vi "CommandInOutTest.vi"() -> ()   [LabVIEW 2014, in "examples.lvlib"]
uses:
  examples.lvlib
  vis/tango_vi.llb/fromDevString.vi
  vis/tango_vi.llb/fromDevVarStringArray.vi
  vis/tango_vi.llb/toDevString.vi
  vis/tango_vi.llb/toDevVarStringArray.vi
  vis/tango_vi.llb/fromDevEnum.vi
  vis/tango_vi.llb/toDevShort.vi
  vis/tango_vi.llb/fromDevUShort.vi
  vis/tango_vi.llb/toDevUShort.vi
  vis/tango_vi.llb/fromDevLong.vi
  vis/tango_vi.llb/toDevLong.vi
  vis/tango_vi.llb/fromDevULong.vi
  vis/tango_vi.llb/toDevULong.vi
  vis/tango_vi.llb/fromDevFloat.vi
  vis/tango_vi.llb/toDevFloat.vi
  vis/tango_vi.llb/fromDevDouble.vi
  vis/tango_vi.llb/toDevDouble.vi
  vis/tango_vi.llb/fromDevVarUShortArray.vi
  vis/tango_vi.llb/toDevVarUShortArray.vi
  vis/tango_vi.llb/fromDevVarULongArray.vi
  vis/tango_vi.llb/toDevVarULongArray.vi
  vis/tango_vi.llb/fromDevVarLongArray.vi
  vis/tango_vi.llb/toDevVarLongArray.vi
  vis/tango_vi.llb/fromDevVarShortArray.vi
  vis/tango_vi.llb/toDevVarShortArray.vi
  vis/tango_vi.llb/fromDevVarFloatArray.vi
  vis/tango_vi.llb/toDevVarFloatArray.vi
  vis/tango_vi.llb/fromDevVarDoubleArray.vi
  vis/tango_vi.llb/toDevVarDoubleArray.vi
  vis/tango_vi.llb/fromDevVarCharArray.vi
  vis/tango_vi.llb/toDevVarCharArray.vi
  vis/tango_vi.llb/fromDevVarDoubleStringArray.vi
  vis/tango_vi.llb/toDevVarDoubleStringArray.vi
  vis/tango_vi.llb/fromDevVarLongStringArray.vi
  vis/tango_vi.llb/toDevVarLongStringArray.vi
  vis/tango_vi.llb/fromDevBoolean.vi
  vis/tango_vi.llb/toDevBoolean.vi
  vis/tango_vi.llb/tango.lvlib
panel:
  out "cmd":bool
  out "Void Example":string="DevBoolean"
  out "Graphe déroulant":i32(graph)
  out "TF example":string="DevBoolean"
  out "cmd":bool
  out "data":bool
  out "Argin":bool
  out "Argout":bool
  out "Argin (svalue)":string[](array[string])
  out "Argin (dvalue)":dbl[](array[numeric])=[0.0, 0.0, 0.0, 0.0, 22.0, 144.0, 108.0, 42.0, 254.0, 232.0, 134.0, 30.0, 230.0, 216.0, 161.0, 246.0, 224.0, 86.0, 234.0, 166.0, 49.0, 58.0, 32.0, 211.0, 173.0, 95.0, 77.0, 181.0, 63.0, 73.0, 167.0, 139.0, 214.0, 190.0, 103.0, 103.0, 169.0, 96.0, 65.0, 97.0, 207.0, 72.0, 125.0, 181.0, 232.0, 13.0, 83.0, 114.0, 134.0, 104.0, 222.0, 186.0, 151.0, 6.0, 244.0, 71.0, 19.0, 16.0, 56.0, 155.0, 85.0, 251.0, 65.0, 85.0, 106.0, 68.0, 170.0, 26.0, 143.0, 0.0, 158.0, 43.0, 118.0, 202.0, 61.0, 68.0, 240.0, 57.0, 209.0, 5.0, 98.0, 217.0, 111.0, 7.0, 202.0, 252.0, 200.0, 153.0, 204.0, 237.0, 228.0, 39.0, 81.0, 253.0, 177.0, 126.0, 199.0, 44.0, 36.0, 175.0, 75.0, 209.0, 178.0, 167.0, 71.0, 225.0, 184.0, 2.0, 157.0, 48.0, 226.0, 233.0, 100.0, 110.0, 187.0, 178.0, 2.0, 135.0, 104.0, 251.0, 131.0, 241.0, 155.0, 13.0, 32.0, 205.0, 77.0, 234.0, 75.0, 144.0, 76.0, 162.0, 196.0, 51.0, 92.0, 150.0, 117.0, 79.0, 178.0, 55.0, 131.0, 128.0, 34.0, 21.0, 93.0, 207.0, 230.0, 166.0, 66.0, 107.0, 39.0, 27.0, 201.0, 85.0, 46.0, 15.0, 57.0, 119.0, 112.0, 178.0, 203.0, 181.0, 186.0, 84.0, 144.0, 207.0, 27.0, 215.0, 81.0, 26.0, 153.0, 210.0, 222.0, 175.0, 212.0, 63.0, 227.0, 175.0, 79.0, 219.0, 119.0, 174.0, 36.0, 214.0, 204.0, 213.0, 83.0, 159.0, 255.0, 63.0, 42.0, 236.0, 74.0, 140.0, 119.0, 3.0, 168.0, 232.0, 161.0, 103.0, 146.0, 193.0, 113.0, 1.0, 139.0, 101.0, 51.0, 131.0, 224.0, 211.0, 244.0, 75.0, 119.0, 231.0, 104.0, 41.0, 169.0, 99.0, 112.0, 204.0, 67.0, 210.0, 99.0, 251.0, 141.0, 239.0, 97.0, 144.0, 211.0, 170.0, 68.0, 6.0, 132.0, 235.0, 191.0, 120.0, 102.0, 48.0, 127.0, 1.0, 97.0, 206.0, 9.0, 103.0, 206.0, 167.0, 249.0, 98.0, 74.0, 193.0, 187.0, 30.0, 113.0, 96.0, 73.0, 61.0]
  out "Argout (svalue)":string[](array[string])
  out "Argout (dvalue)":dbl[](array[numeric])=[0.0, 0.0, 0.0, 0.0, 22.0, 144.0, 108.0, 42.0, 254.0, 232.0, 134.0, 30.0, 230.0, 216.0, 161.0, 246.0, 224.0, 86.0, 234.0, 166.0, 49.0, 58.0, 32.0, 211.0, 173.0, 95.0, 77.0, 181.0, 63.0, 73.0, 167.0, 139.0, 214.0, 190.0, 103.0, 103.0, 169.0, 96.0, 65.0, 97.0, 207.0, 72.0, 125.0, 181.0, 232.0, 13.0, 83.0, 114.0, 134.0, 104.0, 222.0, 186.0, 151.0, 6.0, 244.0, 71.0, 19.0, 16.0, 56.0, 155.0, 85.0, 251.0, 65.0, 85.0, 106.0, 68.0, 170.0, 26.0, 143.0, 0.0, 158.0, 43.0, 118.0, 202.0, 61.0, 68.0, 240.0, 57.0, 209.0, 5.0, 98.0, 217.0, 111.0, 7.0, 202.0, 252.0, 200.0, 153.0, 204.0, 237.0, 228.0, 39.0, 81.0, 253.0, 177.0, 126.0, 199.0, 44.0, 36.0, 175.0, 75.0, 209.0, 178.0, 167.0, 71.0, 225.0, 184.0, 2.0, 157.0, 48.0, 226.0, 233.0, 100.0, 110.0, 187.0, 178.0, 2.0, 135.0, 104.0, 251.0, 131.0, 241.0, 155.0, 13.0, 32.0, 205.0, 77.0, 234.0, 75.0, 144.0, 76.0, 162.0, 196.0, 51.0, 92.0, 150.0, 117.0, 79.0, 178.0, 55.0, 131.0, 128.0, 34.0, 21.0, 93.0, 207.0, 230.0, 166.0, 66.0, 107.0, 39.0, 27.0, 201.0, 85.0, 46.0, 15.0, 57.0, 119.0, 112.0, 178.0, 203.0, 181.0, 186.0, 84.0, 144.0, 207.0, 27.0, 215.0, 81.0, 26.0, 153.0, 210.0, 222.0, 175.0, 212.0, 63.0, 227.0, 175.0, 79.0, 219.0, 119.0, 174.0, 36.0, 214.0, 204.0, 213.0, 83.0, 159.0, 255.0, 63.0, 42.0, 236.0, 74.0, 140.0, 119.0, 3.0, 168.0, 232.0, 161.0, 103.0, 146.0, 193.0, 113.0, 1.0, 139.0, 101.0, 51.0, 131.0, 224.0, 211.0, 244.0, 75.0, 119.0, 231.0, 104.0, 41.0, 169.0, 99.0, 112.0, 204.0, 67.0, 210.0, 99.0, 251.0, 141.0, 239.0, 97.0, 144.0, 211.0, 170.0, 68.0, 6.0, 132.0, 235.0, 191.0, 120.0, 102.0, 48.0, 127.0, 1.0, 97.0, 206.0, 9.0, 103.0, 206.0, 167.0, 249.0, 98.0, 74.0, 193.0, 187.0, 30.0, 113.0, 96.0, 73.0, 61.0]
  out "data":bool
  out "cmd":bool
  out "[DBL][String] example":string="DevVarLongStringArray"
  out "[i32][String] example":string="DevVarLongStringArray"
  out "cmd":bool
  out "data":bool
  out "Argout (lvalue)":i32[](array[numeric])=[0, 0, 0, 0, 22, 144, 108, 42, 254, 232, 134, 30, 230, 216, 161, 246, 224, 86, 234, 166, 49, 58, 32, 211, 173, 95, 77, 181, 63, 73, 167, 139, 214, 190, 103, 103, 169, 96, 65, 97, 207, 72, 125, 181, 232, 13, 83, 114, 134, 104, 222, 186, 151, 6, 244, 71, 19, 16, 56, 155, 85, 251, 65, 85, 106, 68, 170, 26, 143, 0, 158, 43, 118, 202, 61, 68, 240, 57, 209, 5, 98, 217, 111, 7, 202, 252, 200, 153, 204, 237, 228, 39, 81, 253, 177, 126, 199, 44, 36, 175, 75, 209, 178, 167, 71, 225, 184, 2, 157, 48, 226, 233, 100, 110, 187, 178, 2, 135, 104, 251, 131, 241, 155, 13, 32, 205, 77, 234, 75, 144, 76, 162, 196, 51, 92, 150, 117, 79, 178, 55, 131, 128, 34, 21, 93, 207, 230, 166, 66, 107, 39, 27, 201, 85, 46, 15, 57, 119, 112, 178, 203, 181, 186, 84, 144, 207, 27, 215, 81, 26, 153, 210, 222, 175, 212, 63, 227, 175, 79, 219, 119, 174, 36, 214, 204, 213, 83, 159, 255, 63, 42, 236, 74, 140, 119, 3, 168, 232, 161, 103, 146, 193, 113, 1, 139, 101, 51, 131, 224, 211, 244, 75, 119, 231, 104, 41, 169, 99, 112, 204, 67, 210, 99, 251, 141, 239, 97, 144, 211, 170, 68, 6, 132, 235, 191, 120, 102, 48, 127, 1, 97, 206, 9, 103, 206, 167, 249, 98, 74, 193, 187, 30, 113, 96, 73, 61]
  out "Argout (svalue)":string[](array[string])
  out "Argin (lvalue)":i32[](array[numeric])=[0, 0, 0, 0, 22, 144, 108, 42, 254, 232, 134, 30, 230, 216, 161, 246, 224, 86, 234, 166, 49, 58, 32, 211, 173, 95, 77, 181, 63, 73, 167, 139, 214, 190, 103, 103, 169, 96, 65, 97, 207, 72, 125, 181, 232, 13, 83, 114, 134, 104, 222, 186, 151, 6, 244, 71, 19, 16, 56, 155, 85, 251, 65, 85, 106, 68, 170, 26, 143, 0, 158, 43, 118, 202, 61, 68, 240, 57, 209, 5, 98, 217, 111, 7, 202, 252, 200, 153, 204, 237, 228, 39, 81, 253, 177, 126, 199, 44, 36, 175, 75, 209, 178, 167, 71, 225, 184, 2, 157, 48, 226, 233, 100, 110, 187, 178, 2, 135, 104, 251, 131, 241, 155, 13, 32, 205, 77, 234, 75, 144, 76, 162, 196, 51, 92, 150, 117, 79, 178, 55, 131, 128, 34, 21, 93, 207, 230, 166, 66, 107, 39, 27, 201, 85, 46, 15, 57, 119, 112, 178, 203, 181, 186, 84, 144, 207, 27, 215, 81, 26, 153, 210, 222, 175, 212, 63, 227, 175, 79, 219, 119, 174, 36, 214, 204, 213, 83, 159, 255, 63, 42, 236, 74, 140, 119, 3, 168, 232, 161, 103, 146, 193, 113, 1, 139, 101, 51, 131, 224, 211, 244, 75, 119, 231, 104, 41, 169, 99, 112, 204, 67, 210, 99, 251, 141, 239, 97, 144, 211, 170, 68, 6, 132, 235, 191, 120, 102, 48, 127, 1, 97, 206, 9, 103, 206, 167, 249, 98, 74, 193, 187, 30, 113, 96, 73, 61]
  out "Argin (svalue)":string[](array[string])
  out "Argout":string[](array[string])
  out "Argin":string[](array[string])
  out "[String] example":string="DevVarStringArray"
  out "cmd":bool
  out "data":bool
  out "Argout":string
  out "Argin":string
  out "data":bool
  out "cmd":bool
  out "String example":string="DevString"
  out "[u8] example":string="DevVarLongArray"
  out "cmd":bool
  out "Argin":u8[](array[numeric])=[0, 0, 89, 52, 22, 144, 108, 42, 254, 232, 134, 30, 230, 216, 161, 246, 224, 86, 234, 166, 49, 58, 32, 211, 173, 95, 77, 181, 63, 73, 167, 139, 214, 190, 103, 103, 169, 96, 65, 97, 207, 72, 125, 181, 232, 13, 83, 114, 134, 104, 222, 186, 151, 6, 244, 71, 19, 16, 56, 155, 85, 251, 65, 85, 106, 68, 170, 26, 143, 0, 158, 43, 118, 202, 61, 68, 240, 57, 209, 5, 98, 217, 111, 7, 202, 252, 200, 153, 204, 237, 228, 39, 81, 253, 177, 126, 199, 44, 36, 175, 75, 209, 178, 167, 71, 225, 184, 2, 157, 48, 226, 233, 100, 110, 187, 178, 2, 135, 104, 251, 131, 241, 155, 13, 32, 205, 77, 234, 75, 144, 76, 162, 196, 51, 92, 150, 117, 79, 178, 55, 131, 128, 34, 21, 93, 207, 230, 166, 66, 107, 39, 27, 201, 85, 46, 15, 57, 119, 112, 178, 203, 181, 186, 84, 144, 207, 27, 215, 81, 26, 153, 210, 222, 175, 212, 63, 227, 175, 79, 219, 119, 174, 36, 214, 204, 213, 83, 159, 255, 63, 42, 236, 74, 140, 119, 3, 168, 232, 161, 103, 146, 193, 113, 1, 139, 101, 51, 131, 224, 211, 244, 75, 119, 231, 104, 41, 169, 99, 112, 204, 67, 210, 99, 251, 141, 239, 97, 144, 211, 170, 68, 6, 132, 235, 191, 120, 102, 48, 127, 1, 97, 206, 9, 103, 206, 167, 249, 98, 74, 193, 187, 30, 113, 96, 73, 61]
  out "Argout":u8[](array[numeric])=[0, 0, 89, 52, 22, 144, 108, 42, 254, 232, 134, 30, 230, 216, 161, 246, 224, 86, 234, 166, 49, 58, 32, 211, 173, 95, 77, 181, 63, 73, 167, 139, 214, 190, 103, 103, 169, 96, 65, 97, 207, 72, 125, 181, 232, 13, 83, 114, 134, 104, 222, 186, 151, 6, 244, 71, 19, 16, 56, 155, 85, 251, 65, 85, 106, 68, 170, 26, 143, 0, 158, 43, 118, 202, 61, 68, 240, 57, 209, 5, 98, 217, 111, 7, 202, 252, 200, 153, 204, 237, 228, 39, 81, 253, 177, 126, 199, 44, 36, 175, 75, 209, 178, 167, 71, 225, 184, 2, 157, 48, 226, 233, 100, 110, 187, 178, 2, 135, 104, 251, 131, 241, 155, 13, 32, 205, 77, 234, 75, 144, 76, 162, 196, 51, 92, 150, 117, 79, 178, 55, 131, 128, 34, 21, 93, 207, 230, 166, 66, 107, 39, 27, 201, 85, 46, 15, 57, 119, 112, 178, 203, 181, 186, 84, 144, 207, 27, 215, 81, 26, 153, 210, 222, 175, 212, 63, 227, 175, 79, 219, 119, 174, 36, 214, 204, 213, 83, 159, 255, 63, 42, 236, 74, 140, 119, 3, 168, 232, 161, 103, 146, 193, 113, 1, 139, 101, 51, 131, 224, 211, 244, 75, 119, 231, 104, 41, 169, 99, 112, 204, 67, 210, 99, 251, 141, 239, 97, 144, 211, 170, 68, 6, 132, 235, 191, 120, 102, 48, 127, 1, 97, 206, 9, 103, 206, 167, 249, 98, 74, 193, 187, 30, 113, 96, 73, 61]
  out "data":bool
  out "[DBL] example":string="DevVarLongArray"
  out "cmd":bool
  out "Argin":dbl[](array[numeric])=[0.0, 0.0, 89.0, 52.0, 22.0, 144.0, 108.0, 42.0, 254.0, 232.0, 134.0, 30.0, 230.0, 216.0, 161.0, 246.0, 224.0, 86.0, 234.0, 166.0, 49.0, 58.0, 32.0, 211.0, 173.0, 95.0, 77.0, 181.0, 63.0, 73.0, 167.0, 139.0, 214.0, 190.0, 103.0, 103.0, 169.0, 96.0, 65.0, 97.0, 207.0, 72.0, 125.0, 181.0, 232.0, 13.0, 83.0, 114.0, 134.0, 104.0, 222.0, 186.0, 151.0, 6.0, 244.0, 71.0, 19.0, 16.0, 56.0, 155.0, 85.0, 251.0, 65.0, 85.0, 106.0, 68.0, 170.0, 26.0, 143.0, 0.0, 158.0, 43.0, 118.0, 202.0, 61.0, 68.0, 240.0, 57.0, 209.0, 5.0, 98.0, 217.0, 111.0, 7.0, 202.0, 252.0, 200.0, 153.0, 204.0, 237.0, 228.0, 39.0, 81.0, 253.0, 177.0, 126.0, 199.0, 44.0, 36.0, 175.0, 75.0, 209.0, 178.0, 167.0, 71.0, 225.0, 184.0, 2.0, 157.0, 48.0, 226.0, 233.0, 100.0, 110.0, 187.0, 178.0, 2.0, 135.0, 104.0, 251.0, 131.0, 241.0, 155.0, 13.0, 32.0, 205.0, 77.0, 234.0, 75.0, 144.0, 76.0, 162.0, 196.0, 51.0, 92.0, 150.0, 117.0, 79.0, 178.0, 55.0, 131.0, 128.0, 34.0, 21.0, 93.0, 207.0, 230.0, 166.0, 66.0, 107.0, 39.0, 27.0, 201.0, 85.0, 46.0, 15.0, 57.0, 119.0, 112.0, 178.0, 203.0, 181.0, 186.0, 84.0, 144.0, 207.0, 27.0, 215.0, 81.0, 26.0, 153.0, 210.0, 222.0, 175.0, 212.0, 63.0, 227.0, 175.0, 79.0, 219.0, 119.0, 174.0, 36.0, 214.0, 204.0, 213.0, 83.0, 159.0, 255.0, 63.0, 42.0, 236.0, 74.0, 140.0, 119.0, 3.0, 168.0, 232.0, 161.0, 103.0, 146.0, 193.0, 113.0, 1.0, 139.0, 101.0, 51.0, 131.0, 224.0, 211.0, 244.0, 75.0, 119.0, 231.0, 104.0, 41.0, 169.0, 99.0, 112.0, 204.0, 67.0, 210.0, 99.0, 251.0, 141.0, 239.0, 97.0, 144.0, 211.0, 170.0, 68.0, 6.0, 132.0, 235.0, 191.0, 120.0, 102.0, 48.0, 127.0, 1.0, 97.0, 206.0, 9.0, 103.0, 206.0, 167.0, 249.0, 98.0, 74.0, 193.0, 187.0, 30.0, 113.0, 96.0, 73.0, 61.0] format="%#_12g"
  out "Argout":dbl[](array[numeric])=[0.0, 0.0, 89.0, 52.0, 22.0, 144.0, 108.0, 42.0, 254.0, 232.0, 134.0, 30.0, 230.0, 216.0, 161.0, 246.0, 224.0, 86.0, 234.0, 166.0, 49.0, 58.0, 32.0, 211.0, 173.0, 95.0, 77.0, 181.0, 63.0, 73.0, 167.0, 139.0, 214.0, 190.0, 103.0, 103.0, 169.0, 96.0, 65.0, 97.0, 207.0, 72.0, 125.0, 181.0, 232.0, 13.0, 83.0, 114.0, 134.0, 104.0, 222.0, 186.0, 151.0, 6.0, 244.0, 71.0, 19.0, 16.0, 56.0, 155.0, 85.0, 251.0, 65.0, 85.0, 106.0, 68.0, 170.0, 26.0, 143.0, 0.0, 158.0, 43.0, 118.0, 202.0, 61.0, 68.0, 240.0, 57.0, 209.0, 5.0, 98.0, 217.0, 111.0, 7.0, 202.0, 252.0, 200.0, 153.0, 204.0, 237.0, 228.0, 39.0, 81.0, 253.0, 177.0, 126.0, 199.0, 44.0, 36.0, 175.0, 75.0, 209.0, 178.0, 167.0, 71.0, 225.0, 184.0, 2.0, 157.0, 48.0, 226.0, 233.0, 100.0, 110.0, 187.0, 178.0, 2.0, 135.0, 104.0, 251.0, 131.0, 241.0, 155.0, 13.0, 32.0, 205.0, 77.0, 234.0, 75.0, 144.0, 76.0, 162.0, 196.0, 51.0, 92.0, 150.0, 117.0, 79.0, 178.0, 55.0, 131.0, 128.0, 34.0, 21.0, 93.0, 207.0, 230.0, 166.0, 66.0, 107.0, 39.0, 27.0, 201.0, 85.0, 46.0, 15.0, 57.0, 119.0, 112.0, 178.0, 203.0, 181.0, 186.0, 84.0, 144.0, 207.0, 27.0, 215.0, 81.0, 26.0, 153.0, 210.0, 222.0, 175.0, 212.0, 63.0, 227.0, 175.0, 79.0, 219.0, 119.0, 174.0, 36.0, 214.0, 204.0, 213.0, 83.0, 159.0, 255.0, 63.0, 42.0, 236.0, 74.0, 140.0, 119.0, 3.0, 168.0, 232.0, 161.0, 103.0, 146.0, 193.0, 113.0, 1.0, 139.0, 101.0, 51.0, 131.0, 224.0, 211.0, 244.0, 75.0, 119.0, 231.0, 104.0, 41.0, 169.0, 99.0, 112.0, 204.0, 67.0, 210.0, 99.0, 251.0, 141.0, 239.0, 97.0, 144.0, 211.0, 170.0, 68.0, 6.0, 132.0, 235.0, 191.0, 120.0, 102.0, 48.0, 127.0, 1.0, 97.0, 206.0, 9.0, 103.0, 206.0, 167.0, 249.0, 98.0, 74.0, 193.0, 187.0, 30.0, 113.0, 96.0, 73.0, 61.0] format="%#_12g"
  out "data":bool
  out "[SGL] example":string="DevVarLongArray"
  out "cmd":bool
  out "Argin":sgl[](array[numeric])=[0.0, 0.0, 89.0, 52.0, 22.0, 144.0, 108.0, 42.0, 254.0, 232.0, 134.0, 30.0, 230.0, 216.0, 161.0, 246.0, 224.0, 86.0, 234.0, 166.0, 49.0, 58.0, 32.0, 211.0, 173.0, 95.0, 77.0, 181.0, 63.0, 73.0, 167.0, 139.0, 214.0, 190.0, 103.0, 103.0, 169.0, 96.0, 65.0, 97.0, 207.0, 72.0, 125.0, 181.0, 232.0, 13.0, 83.0, 114.0, 134.0, 104.0, 222.0, 186.0, 151.0, 6.0, 244.0, 71.0, 19.0, 16.0, 56.0, 155.0, 85.0, 251.0, 65.0, 85.0, 106.0, 68.0, 170.0, 26.0, 143.0, 0.0, 158.0, 43.0, 118.0, 202.0, 61.0, 68.0, 240.0, 57.0, 209.0, 5.0, 98.0, 217.0, 111.0, 7.0, 202.0, 252.0, 200.0, 153.0, 204.0, 237.0, 228.0, 39.0, 81.0, 253.0, 177.0, 126.0, 199.0, 44.0, 36.0, 175.0, 75.0, 209.0, 178.0, 167.0, 71.0, 225.0, 184.0, 2.0, 157.0, 48.0, 226.0, 233.0, 100.0, 110.0, 187.0, 178.0, 2.0, 135.0, 104.0, 251.0, 131.0, 241.0, 155.0, 13.0, 32.0, 205.0, 77.0, 234.0, 75.0, 144.0, 76.0, 162.0, 196.0, 51.0, 92.0, 150.0, 117.0, 79.0, 178.0, 55.0, 131.0, 128.0, 34.0, 21.0, 93.0, 207.0, 230.0, 166.0, 66.0, 107.0, 39.0, 27.0, 201.0, 85.0, 46.0, 15.0, 57.0, 119.0, 112.0, 178.0, 203.0, 181.0, 186.0, 84.0, 144.0, 207.0, 27.0, 215.0, 81.0, 26.0, 153.0, 210.0, 222.0, 175.0, 212.0, 63.0, 227.0, 175.0, 79.0, 219.0, 119.0, 174.0, 36.0, 214.0, 204.0, 213.0, 83.0, 159.0, 255.0, 63.0, 42.0, 236.0, 74.0, 140.0, 119.0, 3.0, 168.0, 232.0, 161.0, 103.0, 146.0, 193.0, 113.0, 1.0, 139.0, 101.0, 51.0, 131.0, 224.0, 211.0, 244.0, 75.0, 119.0, 231.0, 104.0, 41.0, 169.0, 99.0, 112.0, 204.0, 67.0, 210.0, 99.0, 251.0, 141.0, 239.0, 97.0, 144.0, 211.0, 170.0, 68.0, 6.0, 132.0, 235.0, 191.0, 120.0, 102.0, 48.0, 127.0, 1.0, 97.0, 206.0, 9.0, 103.0, 206.0, 167.0, 249.0, 98.0, 74.0, 193.0, 187.0, 30.0, 113.0, 96.0, 73.0, 61.0]
  out "Argout":sgl[](array[numeric])=[0.0, 0.0, 89.0, 52.0, 22.0, 144.0, 108.0, 42.0, 254.0, 232.0, 134.0, 30.0, 230.0, 216.0, 161.0, 246.0, 224.0, 86.0, 234.0, 166.0, 49.0, 58.0, 32.0, 211.0, 173.0, 95.0, 77.0, 181.0, 63.0, 73.0, 167.0, 139.0, 214.0, 190.0, 103.0, 103.0, 169.0, 96.0, 65.0, 97.0, 207.0, 72.0, 125.0, 181.0, 232.0, 13.0, 83.0, 114.0, 134.0, 104.0, 222.0, 186.0, 151.0, 6.0, 244.0, 71.0, 19.0, 16.0, 56.0, 155.0, 85.0, 251.0, 65.0, 85.0, 106.0, 68.0, 170.0, 26.0, 143.0, 0.0, 158.0, 43.0, 118.0, 202.0, 61.0, 68.0, 240.0, 57.0, 209.0, 5.0, 98.0, 217.0, 111.0, 7.0, 202.0, 252.0, 200.0, 153.0, 204.0, 237.0, 228.0, 39.0, 81.0, 253.0, 177.0, 126.0, 199.0, 44.0, 36.0, 175.0, 75.0, 209.0, 178.0, 167.0, 71.0, 225.0, 184.0, 2.0, 157.0, 48.0, 226.0, 233.0, 100.0, 110.0, 187.0, 178.0, 2.0, 135.0, 104.0, 251.0, 131.0, 241.0, 155.0, 13.0, 32.0, 205.0, 77.0, 234.0, 75.0, 144.0, 76.0, 162.0, 196.0, 51.0, 92.0, 150.0, 117.0, 79.0, 178.0, 55.0, 131.0, 128.0, 34.0, 21.0, 93.0, 207.0, 230.0, 166.0, 66.0, 107.0, 39.0, 27.0, 201.0, 85.0, 46.0, 15.0, 57.0, 119.0, 112.0, 178.0, 203.0, 181.0, 186.0, 84.0, 144.0, 207.0, 27.0, 215.0, 81.0, 26.0, 153.0, 210.0, 222.0, 175.0, 212.0, 63.0, 227.0, 175.0, 79.0, 219.0, 119.0, 174.0, 36.0, 214.0, 204.0, 213.0, 83.0, 159.0, 255.0, 63.0, 42.0, 236.0, 74.0, 140.0, 119.0, 3.0, 168.0, 232.0, 161.0, 103.0, 146.0, 193.0, 113.0, 1.0, 139.0, 101.0, 51.0, 131.0, 224.0, 211.0, 244.0, 75.0, 119.0, 231.0, 104.0, 41.0, 169.0, 99.0, 112.0, 204.0, 67.0, 210.0, 99.0, 251.0, 141.0, 239.0, 97.0, 144.0, 211.0, 170.0, 68.0, 6.0, 132.0, 235.0, 191.0, 120.0, 102.0, 48.0, 127.0, 1.0, 97.0, 206.0, 9.0, 103.0, 206.0, 167.0, 249.0, 98.0, 74.0, 193.0, 187.0, 30.0, 113.0, 96.0, 73.0, 61.0]
  out "data":bool
  out "DBL example":string="DevDouble"
  out "cmd":bool
  out "data":bool
  out "Argin":dbl format="%#_30g"
  out "Argout":dbl format="%#_30g"
  out "SGL example":string="DevFloat"
  out "cmd":bool
  out "data":bool
  out "Argin":sgl
  out "Argout":sgl
  out "u32 example":string="DevULong"
  out "cmd":bool
  out "data":bool
  out "Argin":u32
  out "Argout":u32
  out "i32 example":string="DevLong"
  out "cmd":bool
  out "data":bool
  out "Argin":i32
  out "Argout":i32
  out "Argout":u16
  out "Argin":u16
  out "data":bool
  out "cmd":bool
  out "u16 example":string="DevUShort"
  out "Argout":i16
  out "Argin":i16
  out "data":bool
  out "cmd":bool
  out "i16 example":string="DevShort"
  out "[u32] example":string="DevVarLongArray"
  out "cmd":bool
  out "Argin":i32[](array[numeric])=[0, 0, 89, 52, 22, 144, 108, 42, 254, 232, 134, 30, 230, 216, 161, 246, 224, 86, 234, 166, 49, 58, 32, 211, 173, 95, 77, 181, 63, 73, 167, 139, 214, 190, 103, 103, 169, 96, 65, 97, 207, 72, 125, 181, 232, 13, 83, 114, 134, 104, 222, 186, 151, 6, 244, 71, 19, 16, 56, 155, 85, 251, 65, 85, 106, 68, 170, 26, 143, 0, 158, 43, 118, 202, 61, 68, 240, 57, 209, 5, 98, 217, 111, 7, 202, 252, 200, 153, 204, 237, 228, 39, 81, 253, 177, 126, 199, 44, 36, 175, 75, 209, 178, 167, 71, 225, 184, 2, 157, 48, 226, 233, 100, 110, 187, 178, 2, 135, 104, 251, 131, 241, 155, 13, 32, 205, 77, 234, 75, 144, 76, 162, 196, 51, 92, 150, 117, 79, 178, 55, 131, 128, 34, 21, 93, 207, 230, 166, 66, 107, 39, 27, 201, 85, 46, 15, 57, 119, 112, 178, 203, 181, 186, 84, 144, 207, 27, 215, 81, 26, 153, 210, 222, 175, 212, 63, 227, 175, 79, 219, 119, 174, 36, 214, 204, 213, 83, 159, 255, 63, 42, 236, 74, 140, 119, 3, 168, 232, 161, 103, 146, 193, 113, 1, 139, 101, 51, 131, 224, 211, 244, 75, 119, 231, 104, 41, 169, 99, 112, 204, 67, 210, 99, 251, 141, 239, 97, 144, 211, 170, 68, 6, 132, 235, 191, 120, 102, 48, 127, 1, 97, 206, 9, 103, 206, 167, 249, 98, 74, 193, 187, 30, 113, 96, 73, 61]
  out "Argout":u32[](array[numeric])=[0, 0, 89, 52, 22, 144, 108, 42, 254, 232, 134, 30, 230, 216, 161, 246, 224, 86, 234, 166, 49, 58, 32, 211, 173, 95, 77, 181, 63, 73, 167, 139, 214, 190, 103, 103, 169, 96, 65, 97, 207, 72, 125, 181, 232, 13, 83, 114, 134, 104, 222, 186, 151, 6, 244, 71, 19, 16, 56, 155, 85, 251, 65, 85, 106, 68, 170, 26, 143, 0, 158, 43, 118, 202, 61, 68, 240, 57, 209, 5, 98, 217, 111, 7, 202, 252, 200, 153, 204, 237, 228, 39, 81, 253, 177, 126, 199, 44, 36, 175, 75, 209, 178, 167, 71, 225, 184, 2, 157, 48, 226, 233, 100, 110, 187, 178, 2, 135, 104, 251, 131, 241, 155, 13, 32, 205, 77, 234, 75, 144, 76, 162, 196, 51, 92, 150, 117, 79, 178, 55, 131, 128, 34, 21, 93, 207, 230, 166, 66, 107, 39, 27, 201, 85, 46, 15, 57, 119, 112, 178, 203, 181, 186, 84, 144, 207, 27, 215, 81, 26, 153, 210, 222, 175, 212, 63, 227, 175, 79, 219, 119, 174, 36, 214, 204, 213, 83, 159, 255, 63, 42, 236, 74, 140, 119, 3, 168, 232, 161, 103, 146, 193, 113, 1, 139, 101, 51, 131, 224, 211, 244, 75, 119, 231, 104, 41, 169, 99, 112, 204, 67, 210, 99, 251, 141, 239, 97, 144, 211, 170, 68, 6, 132, 235, 191, 120, 102, 48, 127, 1, 97, 206, 9, 103, 206, 167, 249, 98, 74, 193, 187, 30, 113, 96, 73, 61]
  out "data":bool
  out "data":bool
  out "Argout":u16[](array[numeric])=[0, 0, 89, 52, 22, 144, 108, 42, 254, 232, 134, 30, 230, 216, 161, 246, 224, 86, 234, 166, 49, 58, 32, 211, 173, 95, 77, 181, 63, 73, 167, 139, 214, 190, 103, 103, 169, 96, 65, 97, 207, 72, 125, 181, 232, 13, 83, 114, 134, 104, 222, 186, 151, 6, 244, 71, 19, 16, 56, 155, 85, 251, 65, 85, 106, 68, 170, 26, 143, 0, 158, 43, 118, 202, 61, 68, 240, 57, 209, 5, 98, 217, 111, 7, 202, 252, 200, 153, 204, 237, 228, 39, 81, 253, 177, 126, 199, 44, 36, 175, 75, 209, 178, 167, 71, 225, 184, 2, 157, 48, 226, 233, 100, 110, 187, 178, 2, 135, 104, 251, 131, 241, 155, 13, 32, 205, 77, 234, 75, 144, 76, 162, 196, 51, 92, 150, 117, 79, 178, 55, 131, 128, 34, 21, 93, 207, 230, 166, 66, 107, 39, 27, 201, 85, 46, 15, 57, 119, 112, 178, 203, 181, 186, 84, 144, 207, 27, 215, 81, 26, 153, 210, 222, 175, 212, 63, 227, 175, 79, 219, 119, 174, 36, 214, 204, 213, 83, 159, 255, 63, 42, 236, 74, 140, 119, 3, 168, 232, 161, 103, 146, 193, 113, 1, 139, 101, 51, 131, 224, 211, 244, 75, 119, 231, 104, 41, 169, 99, 112, 204, 67, 210, 99, 251, 141, 239, 97, 144, 211, 170, 68, 6, 132, 235, 191, 120, 102, 48, 127, 1, 97, 206, 9, 103, 206, 167, 249, 98, 74, 193, 187, 30, 113, 96, 73, 61]
  out "Argin":u16[](array[numeric])=[0, 0, 89, 52, 22, 144, 108, 42, 254, 232, 134, 30, 230, 216, 161, 246, 224, 86, 234, 166, 49, 58, 32, 211, 173, 95, 77, 181, 63, 73, 167, 139, 214, 190, 103, 103, 169, 96, 65, 97, 207, 72, 125, 181, 232, 13, 83, 114, 134, 104, 222, 186, 151, 6, 244, 71, 19, 16, 56, 155, 85, 251, 65, 85, 106, 68, 170, 26, 143, 0, 158, 43, 118, 202, 61, 68, 240, 57, 209, 5, 98, 217, 111, 7, 202, 252, 200, 153, 204, 237, 228, 39, 81, 253, 177, 126, 199, 44, 36, 175, 75, 209, 178, 167, 71, 225, 184, 2, 157, 48, 226, 233, 100, 110, 187, 178, 2, 135, 104, 251, 131, 241, 155, 13, 32, 205, 77, 234, 75, 144, 76, 162, 196, 51, 92, 150, 117, 79, 178, 55, 131, 128, 34, 21, 93, 207, 230, 166, 66, 107, 39, 27, 201, 85, 46, 15, 57, 119, 112, 178, 203, 181, 186, 84, 144, 207, 27, 215, 81, 26, 153, 210, 222, 175, 212, 63, 227, 175, 79, 219, 119, 174, 36, 214, 204, 213, 83, 159, 255, 63, 42, 236, 74, 140, 119, 3, 168, 232, 161, 103, 146, 193, 113, 1, 139, 101, 51, 131, 224, 211, 244, 75, 119, 231, 104, 41, 169, 99, 112, 204, 67, 210, 99, 251, 141, 239, 97, 144, 211, 170, 68, 6, 132, 235, 191, 120, 102, 48, 127, 1, 97, 206, 9, 103, 206, 167, 249, 98, 74, 193, 187, 30, 113, 96, 73, 61]
  out "cmd":bool
  out "[u16] example":string="DevVarLongArray"
  out "data":bool
  out "Argout":i16[](array[numeric])=[0, 0, 89, 52, 22, 144, 108, 42, 254, 232, 134, 30, 230, 216, 161, 246, 224, 86, 234, 166, 49, 58, 32, 211, 173, 95, 77, 181, 63, 73, 167, 139, 214, 190, 103, 103, 169, 96, 65, 97, 207, 72, 125, 181, 232, 13, 83, 114, 134, 104, 222, 186, 151, 6, 244, 71, 19, 16, 56, 155, 85, 251, 65, 85, 106, 68, 170, 26, 143, 0, 158, 43, 118, 202, 61, 68, 240, 57, 209, 5, 98, 217, 111, 7, 202, 252, 200, 153, 204, 237, 228, 39, 81, 253, 177, 126, 199, 44, 36, 175, 75, 209, 178, 167, 71, 225, 184, 2, 157, 48, 226, 233, 100, 110, 187, 178, 2, 135, 104, 251, 131, 241, 155, 13, 32, 205, 77, 234, 75, 144, 76, 162, 196, 51, 92, 150, 117, 79, 178, 55, 131, 128, 34, 21, 93, 207, 230, 166, 66, 107, 39, 27, 201, 85, 46, 15, 57, 119, 112, 178, 203, 181, 186, 84, 144, 207, 27, 215, 81, 26, 153, 210, 222, 175, 212, 63, 227, 175, 79, 219, 119, 174, 36, 214, 204, 213, 83, 159, 255, 63, 42, 236, 74, 140, 119, 3, 168, 232, 161, 103, 146, 193, 113, 1, 139, 101, 51, 131, 224, 211, 244, 75, 119, 231, 104, 41, 169, 99, 112, 204, 67, 210, 99, 251, 141, 239, 97, 144, 211, 170, 68, 6, 132, 235, 191, 120, 102, 48, 127, 1, 97, 206, 9, 103, 206, 167, 249, 98, 74, 193, 187, 30, 113, 96, 73, 61]
  out "Argin":i32[](array[numeric])=[0, 0, 89, 52, 22, 144, 108, 42, 254, 232, 134, 30, 230, 216, 161, 246, 224, 86, 234, 166, 49, 58, 32, 211, 173, 95, 77, 181, 63, 73, 167, 139, 214, 190, 103, 103, 169, 96, 65, 97, 207, 72, 125, 181, 232, 13, 83, 114, 134, 104, 222, 186, 151, 6, 244, 71, 19, 16, 56, 155, 85, 251, 65, 85, 106, 68, 170, 26, 143, 0, 158, 43, 118, 202, 61, 68, 240, 57, 209, 5, 98, 217, 111, 7, 202, 252, 200, 153, 204, 237, 228, 39, 81, 253, 177, 126, 199, 44, 36, 175, 75, 209, 178, 167, 71, 225, 184, 2, 157, 48, 226, 233, 100, 110, 187, 178, 2, 135, 104, 251, 131, 241, 155, 13, 32, 205, 77, 234, 75, 144, 76, 162, 196, 51, 92, 150, 117, 79, 178, 55, 131, 128, 34, 21, 93, 207, 230, 166, 66, 107, 39, 27, 201, 85, 46, 15, 57, 119, 112, 178, 203, 181, 186, 84, 144, 207, 27, 215, 81, 26, 153, 210, 222, 175, 212, 63, 227, 175, 79, 219, 119, 174, 36, 214, 204, 213, 83, 159, 255, 63, 42, 236, 74, 140, 119, 3, 168, 232, 161, 103, 146, 193, 113, 1, 139, 101, 51, 131, 224, 211, 244, 75, 119, 231, 104, 41, 169, 99, 112, 204, 67, 210, 99, 251, 141, 239, 97, 144, 211, 170, 68, 6, 132, 235, 191, 120, 102, 48, 127, 1, 97, 206, 9, 103, 206, 167, 249, 98, 74, 193, 187, 30, 113, 96, 73, 61]
  out "cmd":bool
  out "[i16] example":string="DevVarLongArray"
  out "data":bool
  out "Argout":i32[](array[numeric])=[0, 0, 89, 52, 22, 144, 108, 42, 254, 232, 134, 30, 230, 216, 161, 246, 224, 86, 234, 166, 49, 58, 32, 211, 173, 95, 77, 181, 63, 73, 167, 139, 214, 190, 103, 103, 169, 96, 65, 97, 207, 72, 125, 181, 232, 13, 83, 114, 134, 104, 222, 186, 151, 6, 244, 71, 19, 16, 56, 155, 85, 251, 65, 85, 106, 68, 170, 26, 143, 0, 158, 43, 118, 202, 61, 68, 240, 57, 209, 5, 98, 217, 111, 7, 202, 252, 200, 153, 204, 237, 228, 39, 81, 253, 177, 126, 199, 44, 36, 175, 75, 209, 178, 167, 71, 225, 184, 2, 157, 48, 226, 233, 100, 110, 187, 178, 2, 135, 104, 251, 131, 241, 155, 13, 32, 205, 77, 234, 75, 144, 76, 162, 196, 51, 92, 150, 117, 79, 178, 55, 131, 128, 34, 21, 93, 207, 230, 166, 66, 107, 39, 27, 201, 85, 46, 15, 57, 119, 112, 178, 203, 181, 186, 84, 144, 207, 27, 215, 81, 26, 153, 210, 222, 175, 212, 63, 227, 175, 79, 219, 119, 174, 36, 214, 204, 213, 83, 159, 255, 63, 42, 236, 74, 140, 119, 3, 168, 232, 161, 103, 146, 193, 113, 1, 139, 101, 51, 131, 224, 211, 244, 75, 119, 231, 104, 41, 169, 99, 112, 204, 67, 210, 99, 251, 141, 239, 97, 144, 211, 170, 68, 6, 132, 235, 191, 120, 102, 48, 127, 1, 97, 206, 9, 103, 206, 167, 249, 98, 74, 193, 187, 30, 113, 96, 73, 61]
  out "Argin":i32[](array[numeric])=[0, 0, 89, 52, 22, 144, 108, 42, 254, 232, 134, 30, 230, 216, 161, 246, 224, 86, 234, 166, 49, 58, 32, 211, 173, 95, 77, 181, 63, 73, 167, 139, 214, 190, 103, 103, 169, 96, 65, 97, 207, 72, 125, 181, 232, 13, 83, 114, 134, 104, 222, 186, 151, 6, 244, 71, 19, 16, 56, 155, 85, 251, 65, 85, 106, 68, 170, 26, 143, 0, 158, 43, 118, 202, 61, 68, 240, 57, 209, 5, 98, 217, 111, 7, 202, 252, 200, 153, 204, 237, 228, 39, 81, 253, 177, 126, 199, 44, 36, 175, 75, 209, 178, 167, 71, 225, 184, 2, 157, 48, 226, 233, 100, 110, 187, 178, 2, 135, 104, 251, 131, 241, 155, 13, 32, 205, 77, 234, 75, 144, 76, 162, 196, 51, 92, 150, 117, 79, 178, 55, 131, 128, 34, 21, 93, 207, 230, 166, 66, 107, 39, 27, 201, 85, 46, 15, 57, 119, 112, 178, 203, 181, 186, 84, 144, 207, 27, 215, 81, 26, 153, 210, 222, 175, 212, 63, 227, 175, 79, 219, 119, 174, 36, 214, 204, 213, 83, 159, 255, 63, 42, 236, 74, 140, 119, 3, 168, 232, 161, 103, 146, 193, 113, 1, 139, 101, 51, 131, 224, 211, 244, 75, 119, 231, 104, 41, 169, 99, 112, 204, 67, 210, 99, 251, 141, 239, 97, 144, 211, 170, 68, 6, 132, 235, 191, 120, 102, 48, 127, 1, 97, 206, 9, 103, 206, 167, 249, 98, 74, 193, 187, 30, 113, 96, 73, 61]
  out "cmd":bool
  out "[I32] example":string="DevVarLongArray"
  out "alive":bool
  out "State Color":u32(colorbox)=16448250
  out "Status":string
  out "State String":string
  out "State Code":i16
  in  "TangoTest Device Name":string="sys/tg_test/1"
  # "TANGO  Binding for LabVIEW - Command I/O example"
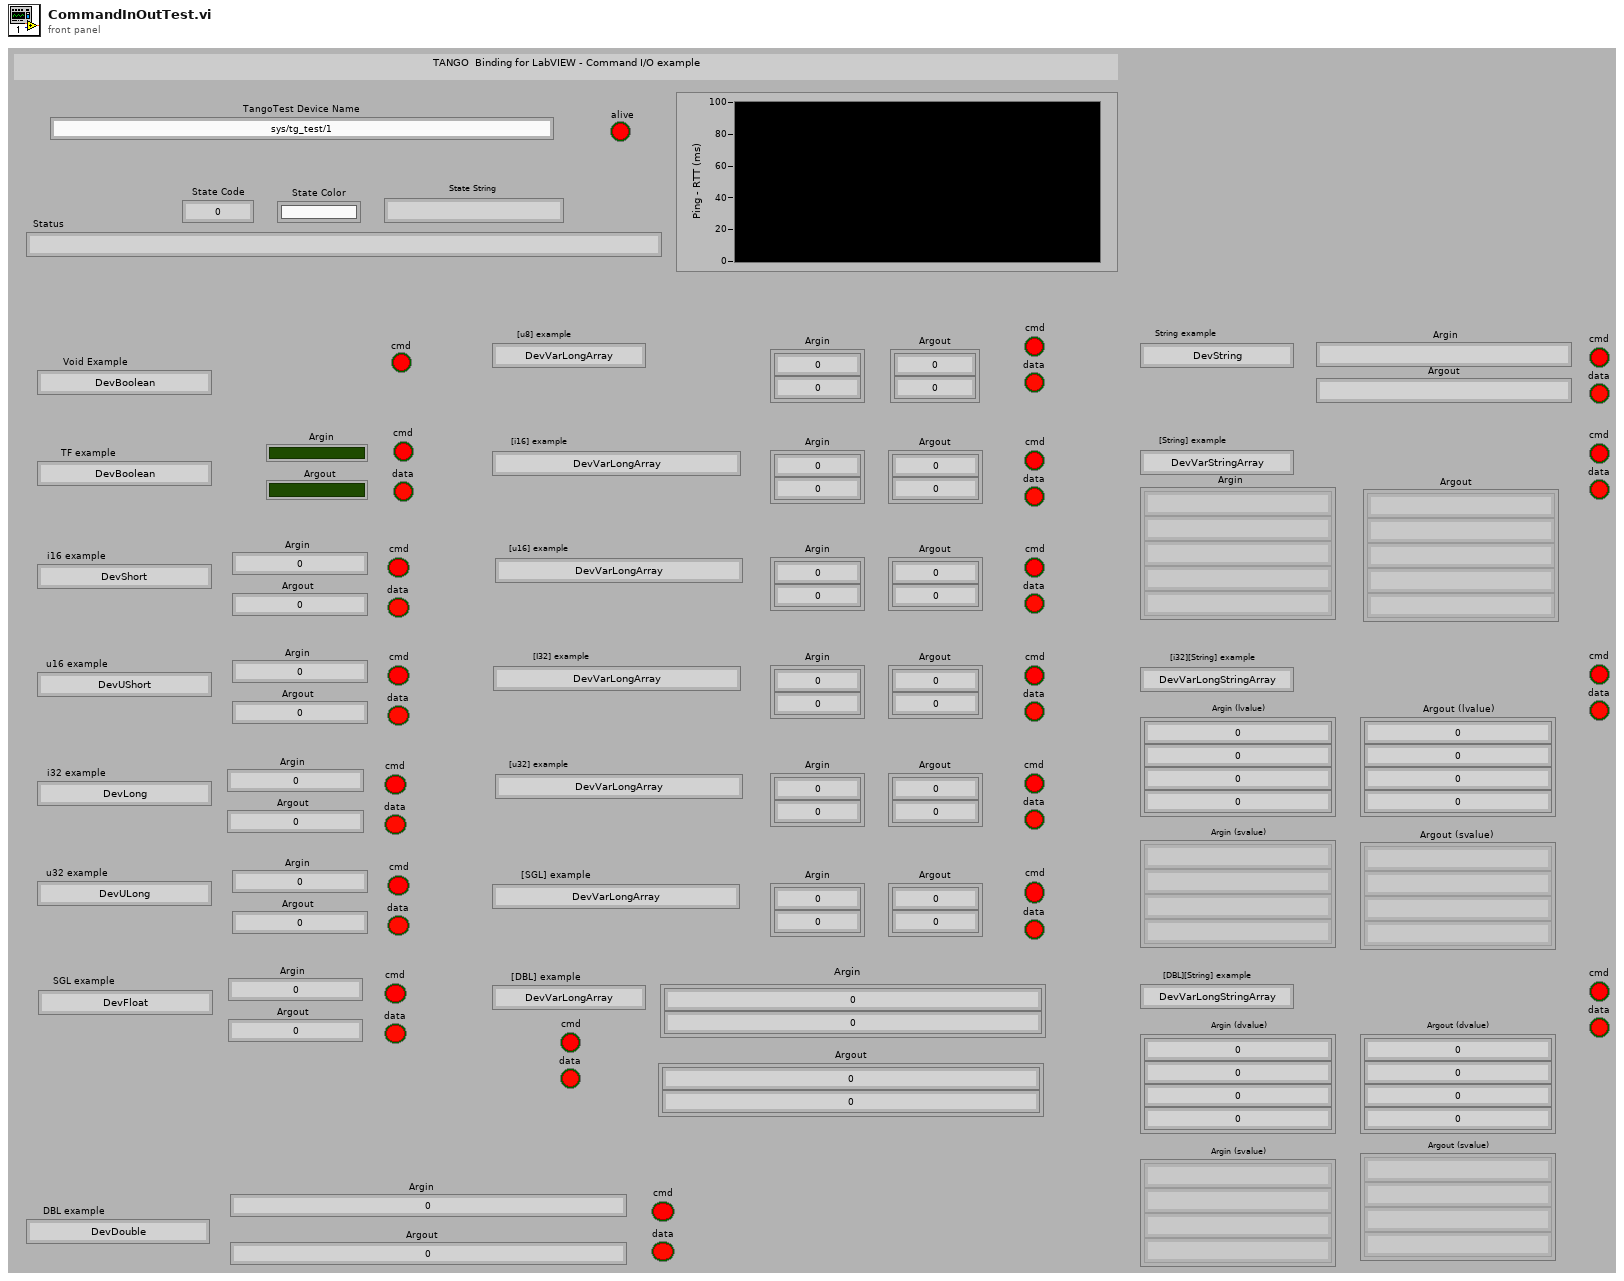
[diagram p1: front panel]
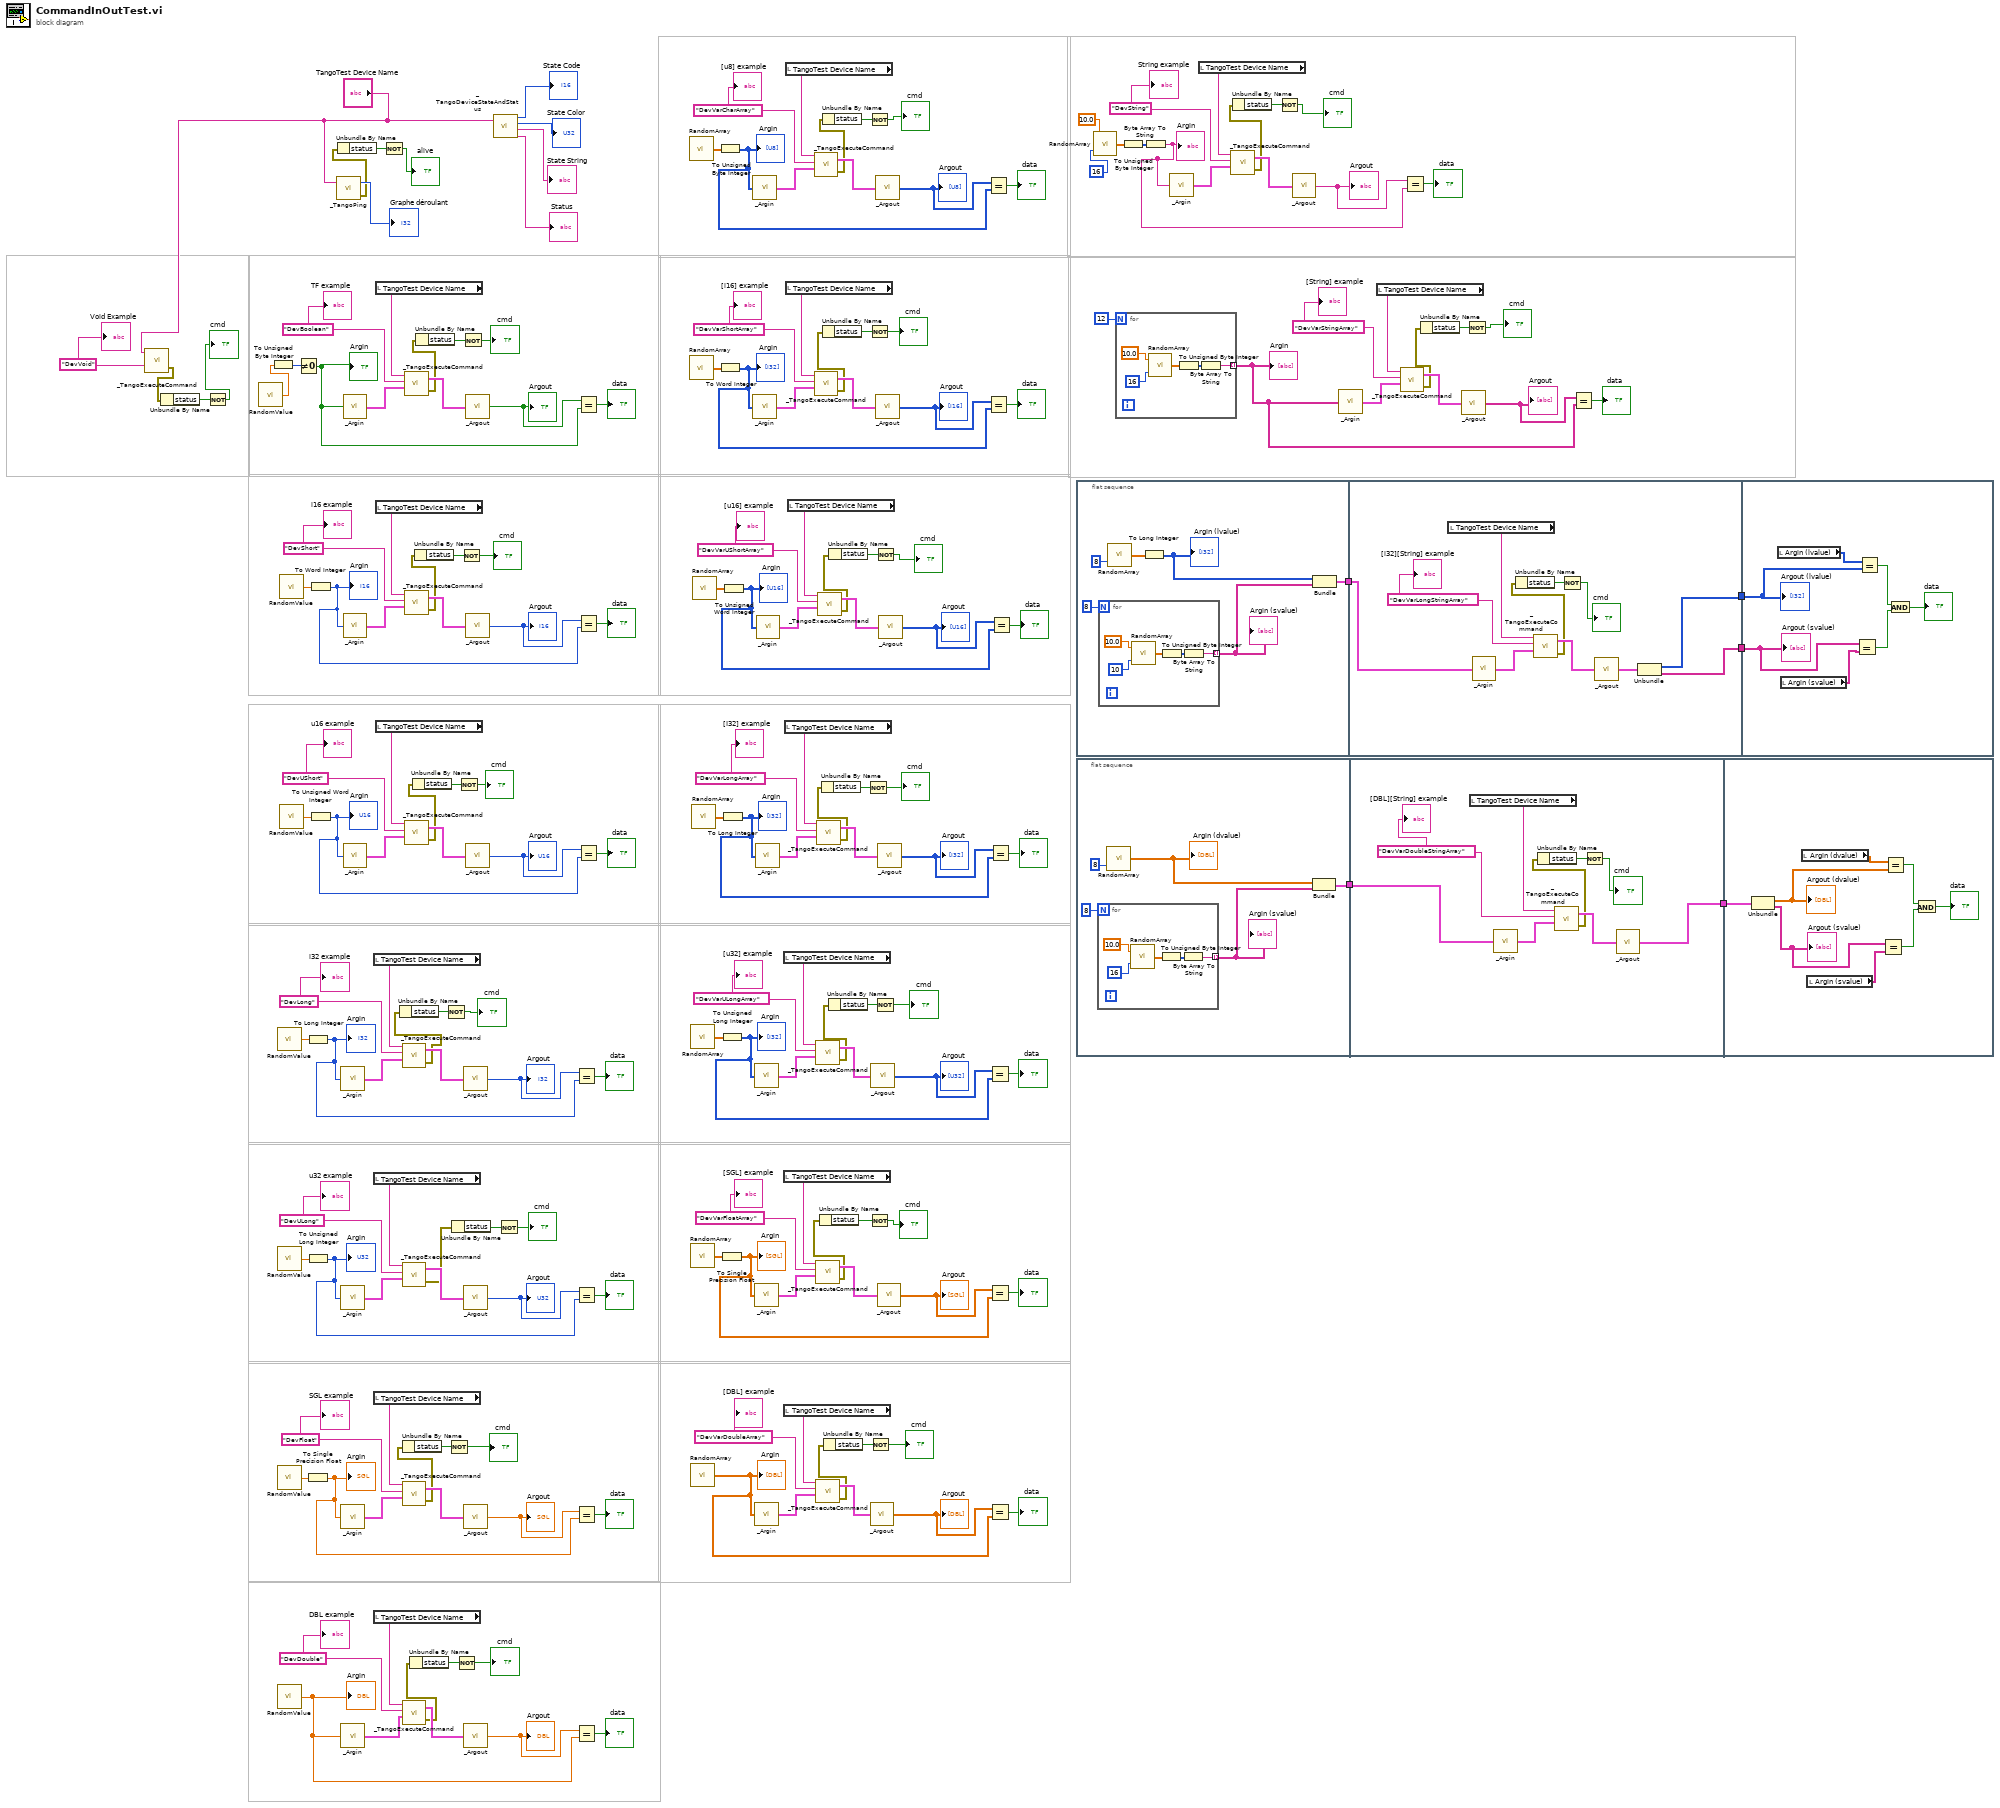
[diagram p0: block diagram]
diagram:
  w59 = "DevVoid"
  w70 = "DevBoolean"
  w80 = "DevVarStringArray"
  w88 = "DevVarCharArray"
  w98 = "DevVarDoubleArray"
  w107 = "DevVarFloatArray"
  w113 = "DevDouble"
  w116 = "DevFloat"
  w127 = "DevULong"
  w133 = "DevLong"
  w144 = "DevUShort"
  w152 = "DevShort"
  w157 = "DevVarULongArray"
  w168 = "DevVarUShortArray"
  w176 = "DevVarShortArray"
  w182 = "DevString"
  w190 = "DevVarLongArray"
  n1 = call "_TangoExecuteCommand.vi"("command name"=w59, "device name"="TangoTest Device Name") -> ("error out"=w52:errorcluster)  [unwired: 2 in, 1 out]
  n2 = Unbundle By Name(w52) -> ("status"=w53:bool)
  n3 = Not(x=w53) -> (.not. x?=→"cmd":bool)
  n4 = call "RandomValue.vi"() -> ("random value"=w1:dbl)  [unwired: 1 in]
  n5 = To Unsigned Byte Integer(number=w1) -> (unsigned 8bit integer=w67:u8)
  n6 = call "RandomValue.vi"() -> ("random value"=w135:dbl)  [unwired: 1 in]
  n7 = call "RandomValue.vi"() -> ("random value"=w125:dbl)  [unwired: 1 in]
  n8 = call "RandomValue.vi"() -> ("random value"=w118:dbl)  [unwired: 1 in]
  n9 = call "RandomValue.vi"() -> ("random value"=w2:dbl)  [unwired: 1 in]
  "Argin" <- w2
  n10 = call "RandomValue.vi"() -> ("random value"=w150:dbl)  [unwired: 1 in]
  n11 = call "RandomValue.vi"() -> ("random value"=w142:dbl)  [unwired: 1 in]
  n12 = Not Equal To 0?(x=w67) -> (x != 0?=w66:bool)
  "Argin" <- w66
  n13 = To Long Integer(number=w135) -> (32bit integer=w138:i32)
  "Argin" <- w138
  n14 = To Unsigned Long Integer(number=w125) -> (unsigned 32bit integer=w122:u32)
  "Argin" <- w122
  n15 = To Single Precision Float(number=w118) -> (single precision float=w121:sgl)
  "Argin" <- w121
  n16 = To Word Integer(number=w150) -> (16bit integer=w148:i16)
  "Argin" <- w148
  n17 = To Unsigned Word Integer(number=w142) -> (unsigned 16bit integer=w139:u16)
  "Argin" <- w139
  n18 = call "_TangoPing.vi"("device name"="TangoTest Device Name") -> ("error out"=w4:errorcluster, "rrt"=→"Graphe déroulant":i32)  [unwired: 1 in]
  n19 = Unbundle By Name(w4) -> ("status"=w5:bool)
  n20 = call-poly "_Argin.vi"("argin"=w138) -> ("ArgIO"=w131:cluster{"num data":u8[], "str data":string[]})
  n21 = call-poly "_Argin.vi"("argin"=w122) -> ("ArgIO"=w130:cluster{"num data":u8[], "str data":string[]})
  n22 = call-poly "_Argin.vi"("argin"=w121) -> ("ArgIO"=w114:cluster{"num data":u8[], "str data":string[]})
  n23 = call-poly "_Argin.vi"("argin"=w2) -> ("ArgIO"=w57:cluster{"num data":u8[], "str data":string[]})
  n24 = call-poly "_Argin.vi"("argin"=w66) -> ("ArgIO"=w68:cluster{"num data":u8[], "str data":string[]})
  n25 = call-poly "_Argin.vi"("argin"=w148) -> ("ArgIO"=w154:cluster{"num data":u8[], "str data":string[]})
  n26 = call-poly "_Argin.vi"("argin"=w139) -> ("ArgIO"=w146:cluster{"num data":u8[], "str data":string[]})
  n27 = local read "TangoTest Device Name"() -> (w134:string)
  n28 = local read "TangoTest Device Name"() -> (w126:string)
  n29 = local read "TangoTest Device Name"() -> (w117:string)
  n30 = local read "TangoTest Device Name"() -> (w112:string)
  n31 = local read "TangoTest Device Name"() -> (w71:string)
  n32 = local read "TangoTest Device Name"() -> (w151:string)
  n33 = local read "TangoTest Device Name"() -> (w143:string)
  n34 = Not(x=w5) -> (.not. x?=→"alive":bool)
  n35 = call "_TangoExecuteCommand.vi"("argin"=w131, "command name"=w133, "device name"=w134) -> ("error out"=w39:errorcluster, "argout"=w132:cluster{"num data":u8[], "str data":string[]})  [unwired: 1 in]
  n36 = Unbundle By Name(w39) -> ("status"=w41:bool)
  n37 = call "_TangoExecuteCommand.vi"("argin"=w130, "command name"=w127, "device name"=w126) -> ("error out"=w128:errorcluster, "argout"=w129:cluster{"num data":u8[], "str data":string[]})  [unwired: 1 in]
  n38 = call "_TangoExecuteCommand.vi"("argin"=w114, "command name"=w116, "device name"=w117) -> ("error out"=w36:errorcluster, "argout"=w115:cluster{"num data":u8[], "str data":string[]})  [unwired: 1 in]
  n39 = Unbundle By Name(w36) -> ("status"=w38:bool)
  n40 = call "_TangoExecuteCommand.vi"("argin"=w57, "command name"=w113, "device name"=w112) -> ("error out"=w33:errorcluster, "argout"=w56:cluster{"num data":u8[], "str data":string[]})  [unwired: 1 in]
  n41 = call "_TangoExecuteCommand.vi"("argin"=w68, "command name"=w70, "device name"=w71) -> ("error out"=w48:errorcluster, "argout"=w69:cluster{"num data":u8[], "str data":string[]})  [unwired: 1 in]
  n42 = call "_TangoExecuteCommand.vi"("argin"=w154, "command name"=w152, "device name"=w151) -> ("error out"=w45:errorcluster, "argout"=w153:cluster{"num data":u8[], "str data":string[]})  [unwired: 1 in]
  n43 = call "_TangoExecuteCommand.vi"("argin"=w146, "command name"=w144, "device name"=w143) -> ("error out"=w42:errorcluster, "argout"=w145:cluster{"num data":u8[], "str data":string[]})  [unwired: 1 in]
  n44 = Unbundle By Name(w33) -> ("status"=w35:bool)
  n45 = Unbundle By Name(w42) -> ("status"=w44:bool)
  n46 = Unbundle By Name(w45) -> ("status"=w47:bool)
  n47 = Unbundle By Name(w48) -> ("status"=w50:bool)
  n48 = Not(x=w41) -> (.not. x?=→"cmd":bool)
  n49 = Not(x=w38) -> (.not. x?=→"cmd":bool)
  n50 = Unbundle By Name(w128) -> ("status"=w55:bool)
  n51 = Not(x=w35) -> (.not. x?=→"cmd":bool)
  n52 = Not(x=w44) -> (.not. x?=→"cmd":bool)
  n53 = Not(x=w47) -> (.not. x?=→"cmd":bool)
  n54 = Not(x=w50) -> (.not. x?=→"cmd":bool)
  n55 = call-poly "_Argout.vi"("ArgIO"=w132) -> ("argout"=w137:i32)
  "Argout" <- w137
  n56 = call-poly "_Argout.vi"("ArgIO"=w129) -> ("argout"=w123:u32)
  "Argout" <- w123
  n57 = call-poly "_Argout.vi"("ArgIO"=w115) -> ("argout"=w120:sgl)
  "Argout" <- w120
  n58 = call-poly "_Argout.vi"("ArgIO"=w56) -> ("argout"=w110:dbl)
  "Argout" <- w110
  n59 = call-poly "_Argout.vi"("ArgIO"=w69) -> ("argout"=w73:bool)
  "Argout" <- w73
  n60 = call-poly "_Argout.vi"("ArgIO"=w153) -> ("argout"=w147:i16)
  "Argout" <- w147
  n61 = call-poly "_Argout.vi"("ArgIO"=w145) -> ("argout"=w140:u16)
  "Argout" <- w140
  n62 = call "_TangoDeviceStateAndStatus.vi"("Device Name"="TangoTest Device Name") -> ("Status"=→"Status":string, "State String"=→"State String":string, "State Color"=→"State Color":u32, "State Code"=→"State Code":i16)  [unwired: 1 in, 1 out]
  n63 = Not(x=w55) -> (.not. x?=→"cmd":bool)
  n64 = Equal?(x=w137, y=w138) -> (x = y?=→"data":bool)
  n65 = Equal?(x=w123, y=w122) -> (x = y?=→"data":bool)
  n66 = Equal?(x=w120, y=w121) -> (x = y?=→"data":bool)
  n67 = Equal?(x=w110, y=w2) -> (x = y?=→"data":bool)
  n68 = Equal?(x=w73, y=w66) -> (x = y?=→"data":bool)
  n69 = Equal?(x=w147, y=w148) -> (x = y?=→"data":bool)
  n70 = Equal?(x=w140, y=w139) -> (x = y?=→"data":bool)
  n71 = call "RandomArray.vi"() -> ("random array"=w90:dbl[])  [unwired: 2 in]
  n72 = call "RandomArray.vi"() -> ("random array"=w174:dbl[])  [unwired: 2 in]
  n73 = call "RandomArray.vi"() -> ("random array"=w159:dbl[])  [unwired: 2 in]
  n74 = call "RandomArray.vi"() -> ("random array"=w105:dbl[])  [unwired: 2 in]
  n75 = call "RandomArray.vi"() -> ("random array"=w95:dbl[])  [unwired: 2 in]
  "Argin" <- w95
  n76 = call "RandomArray.vi"() -> ("random array"=w188:dbl[])  [unwired: 2 in]
  n77 = call "RandomArray.vi"() -> ("random array"=w166:dbl[])  [unwired: 2 in]
  n78 = To Unsigned Byte Integer(number=w90) -> (unsigned 8bit integer=w91:u8[])
  "Argin" <- w91
  n79 = To Word Integer(number=w174) -> (16bit integer=w173:i16[])
  "Argin" <- w173
  n80 = To Unsigned Long Integer(number=w159) -> (unsigned 32bit integer=w160:u32[])
  "Argin" <- w160
  n81 = To Single Precision Float(number=w105) -> (single precision float=w104:sgl[])
  "Argin" <- w104
  n82 = To Long Integer(number=w188) -> (32bit integer=w187:i32[])
  "Argin" <- w187
  n83 = To Unsigned Word Integer(number=w166) -> (unsigned 16bit integer=w165:u16[])
  "Argin" <- w165
  n84 = call-poly "_Argin.vi"("argin"=w91) -> ("ArgIO"=w87:cluster{"num data":u8[], "str data":string[]})
  n85 = call-poly "_Argin.vi"("argin"=w173) -> ("ArgIO"=w178:cluster{"num data":u8[], "str data":string[]})
  n86 = call-poly "_Argin.vi"("argin"=w160) -> ("ArgIO"=w155:cluster{"num data":u8[], "str data":string[]})
  n87 = call-poly "_Argin.vi"("argin"=w104) -> ("ArgIO"=w109:cluster{"num data":u8[], "str data":string[]})
  n88 = call-poly "_Argin.vi"("argin"=w95) -> ("ArgIO"=w96:cluster{"num data":u8[], "str data":string[]})
  n89 = call-poly "_Argin.vi"("argin"=w187) -> ("ArgIO"=w192:cluster{"num data":u8[], "str data":string[]})
  n90 = call-poly "_Argin.vi"("argin"=w165) -> ("ArgIO"=w170:cluster{"num data":u8[], "str data":string[]})
  n91 = local read "TangoTest Device Name"() -> (w158:string)
  n92 = local read "TangoTest Device Name"() -> (w106:string)
  n93 = local read "TangoTest Device Name"() -> (w99:string)
  n94 = local read "TangoTest Device Name"() -> (w189:string)
  n95 = local read "TangoTest Device Name"() -> (w89:string)
  n96 = local read "TangoTest Device Name"() -> (w175:string)
  n97 = local read "TangoTest Device Name"() -> (w167:string)
  n98 = call "_TangoExecuteCommand.vi"("argin"=w87, "command name"=w88, "device name"=w89) -> ("error out"=w12:errorcluster, "argout"=w60:cluster{"num data":u8[], "str data":string[]})  [unwired: 1 in]
  n99 = call "_TangoExecuteCommand.vi"("argin"=w178, "command name"=w176, "device name"=w175) -> ("error out"=w15:errorcluster, "argout"=w177:cluster{"num data":u8[], "str data":string[]})  [unwired: 1 in]
  n100 = call "_TangoExecuteCommand.vi"("argin"=w155, "command name"=w157, "device name"=w158) -> ("error out"=w24:errorcluster, "argout"=w156:cluster{"num data":u8[], "str data":string[]})  [unwired: 1 in]
  n101 = call "_TangoExecuteCommand.vi"("argin"=w109, "command name"=w107, "device name"=w106) -> ("error out"=w27:errorcluster, "argout"=w108:cluster{"num data":u8[], "str data":string[]})  [unwired: 1 in]
  n102 = call "_TangoExecuteCommand.vi"("argin"=w96, "command name"=w98, "device name"=w99) -> ("error out"=w30:errorcluster, "argout"=w97:cluster{"num data":u8[], "str data":string[]})  [unwired: 1 in]
  n103 = call "_TangoExecuteCommand.vi"("argin"=w192, "command name"=w190, "device name"=w189) -> ("error out"=w21:errorcluster, "argout"=w191:cluster{"num data":u8[], "str data":string[]})  [unwired: 1 in]
  n104 = call "_TangoExecuteCommand.vi"("argin"=w170, "command name"=w168, "device name"=w167) -> ("error out"=w19:errorcluster, "argout"=w169:cluster{"num data":u8[], "str data":string[]})  [unwired: 1 in]
  n105 = Unbundle By Name(w27) -> ("status"=w29:bool)
  n106 = Unbundle By Name(w21) -> ("status"=w23:bool)
  n107 = Unbundle By Name(w12) -> ("status"=w14:bool)
  n108 = Unbundle By Name(w15) -> ("status"=w17:bool)
  n109 = Unbundle By Name(w30) -> ("status"=w32:bool)
  n110 = Unbundle By Name(w24) -> ("status"=w26:bool)
  n111 = Unbundle By Name(w19) -> ("status"=w20:bool)
  n112 = Not(x=w23) -> (.not. x?=→"cmd":bool)
  n113 = Not(x=w14) -> (.not. x?=→"cmd":bool)
  n114 = Not(x=w17) -> (.not. x?=→"cmd":bool)
  n115 = Not(x=w29) -> (.not. x?=→"cmd":bool)
  n116 = Not(x=w32) -> (.not. x?=→"cmd":bool)
  n117 = call-poly "_Argout.vi"("ArgIO"=w97) -> ("argout"=w100:dbl[])
  "Argout" <- w100
  n118 = call-poly "_Argout.vi"("ArgIO"=w156) -> ("argout"=w161:u32[])
  "Argout" <- w161
  n119 = Not(x=w26) -> (.not. x?=→"cmd":bool)
  n120 = Not(x=w20) -> (.not. x?=→"cmd":bool)
  n121 = call-poly "_Argout.vi"("ArgIO"=w60) -> ("argout"=w92:u8[])
  "Argout" <- w92
  n122 = call-poly "_Argout.vi"("ArgIO"=w177) -> ("argout"=w172:i16[])
  "Argout" <- w172
  n123 = call-poly "_Argout.vi"("ArgIO"=w108) -> ("argout"=w103:sgl[])
  "Argout" <- w103
  n124 = call-poly "_Argout.vi"("ArgIO"=w191) -> ("argout"=w186:i32[])
  "Argout" <- w186
  n125 = call-poly "_Argout.vi"("ArgIO"=w169) -> ("argout"=w164:u16[])
  "Argout" <- w164
  n126 = Equal?(x=w92, y=w91) -> (x = y?=→"data":bool)
  n127 = Equal?(x=w172, y=w173) -> (x = y?=→"data":bool)
  n128 = Equal?(x=w161, y=w160) -> (x = y?=→"data":bool)
  n129 = Equal?(x=w103, y=w104) -> (x = y?=→"data":bool)
  n130 = Equal?(x=w100, y=w95) -> (x = y?=→"data":bool)
  n131 = Equal?(x=w186, y=w187) -> (x = y?=→"data":bool)
  n132 = Equal?(x=w164, y=w165) -> (x = y?=→"data":bool)
  n133 = flat-sequence {
    tunnel: [w197] -> w65
    tunnel: w65 -> [w212]
    tunnel: [w211] -> w64
    tunnel: w64 -> [w217]
    frame #0 {
      n134 = for {
        N: 8 -> [_]
        tunnel: [w202] -> w198 mode=indexing
        n135 = call "RandomArray.vi"("random array size"=16, "factor"=10.0) -> ("random array"=w206:dbl[])
        n136 = To Unsigned Byte Integer(number=w206) -> (unsigned 8bit integer=w205:u8[])
        n137 = Byte Array To String(unsigned byte array=w205) -> (string=w202:string)
      }
      "Argin (svalue)" <- w198
      n138 = call "RandomArray.vi"("random array size"=8) -> ("random array"=w200:dbl[])  [unwired: 1 in]
      "Argin (dvalue)" <- w200
      n139 = Bundle("random array"=w200, w198) -> (w197:cluster{"random array":dbl[], string[]})  [unwired: 1 in]
    }
    frame #1 {
      w210 = "DevVarDoubleStringArray"
      n140 = local read "TangoTest Device Name"() -> (w215:string)
      n141 = call-poly "_Argin.vi"("argin"=w212) -> ("ArgIO"=w213:cluster{"num data":u8[], "str data":string[]})
      n142 = call "_TangoExecuteCommand.vi"("argin"=w213, "command name"=w210, "device name"=w215) -> ("error out"=w207:errorcluster, "argout"=w214:cluster{"num data":u8[], "str data":string[]})  [unwired: 1 in]
      n143 = Unbundle By Name(w207) -> ("status"=w209:bool)
      n144 = Not(x=w209) -> (.not. x?=→"cmd":bool)
      n145 = call-poly "_Argout.vi"("ArgIO"=w214) -> ("argout"=w211:cluster{"dvalue":dbl[], "svalue":string[]})
      "[DBL][String] example" <- w210
    }
    frame #2 {
      n146 = Unbundle(w217) -> ("dvalue"=w220:dbl[], "svalue"=w216:string[])
      "Argout (svalue)" <- w216
      "Argout (dvalue)" <- w220
      n147 = local read "Argin (dvalue)"() -> (w219:dbl[])
      n148 = local read "Argin (svalue)"() -> (w218:string[])
      n149 = Equal?(x=w216, y=w218) -> (x = y?=w223:bool)
      n150 = Equal?(x=w219, y=w220) -> (x = y?=w222:bool)
      n151 = And(x=w222, y=w223) -> (x .and. y?=→"data":bool)
    }
  }
  n152 = flat-sequence {
    tunnel: [w224] -> w61
    tunnel: [w240] -> w63
    tunnel: [w239] -> w62
    tunnel: w61 -> [w238]
    tunnel: w63 -> [w246]
    tunnel: w62 -> [w247]
    frame #0 {
      n153 = for {
        N: 8 -> [_]
        tunnel: [w230] -> w227 mode=indexing
        n154 = call "RandomArray.vi"("random array size"=10, "factor"=10.0) -> ("random array"=w234:dbl[])
        n155 = To Unsigned Byte Integer(number=w234) -> (unsigned 8bit integer=w233:u8[])
        n156 = Byte Array To String(unsigned byte array=w233) -> (string=w230:string)
      }
      "Argin (svalue)" <- w227
      n157 = call "RandomArray.vi"("random array size"=8) -> ("random array"=w226:dbl[])  [unwired: 1 in]
      n158 = To Long Integer(number=w226) -> (32bit integer=w228:i32[])
      "Argin (lvalue)" <- w228
      n159 = Bundle(w228, w227) -> (w224:cluster{i32[], string[]})  [unwired: 1 in]
    }
    frame #1 {
      w243 = "DevVarLongStringArray"
      n160 = local read "TangoTest Device Name"() -> (w242:string)
      n161 = call-poly "_Argin.vi"("argin"=w238) -> ("ArgIO"=w245:cluster{"num data":u8[], "str data":string[]})
      n162 = call "_TangoExecuteCommand.vi"("argin"=w245, "command name"=w243, "device name"=w242) -> ("error out"=w235:errorcluster, "argout"=w244:cluster{"num data":u8[], "str data":string[]})  [unwired: 1 in]
      n163 = Unbundle By Name(w235) -> ("status"=w237:bool)
      n164 = Not(x=w237) -> (.not. x?=→"cmd":bool)
      n165 = call-poly "_Argout.vi"("ArgIO"=w244) -> ("argout"=w241:cluster{"lvalue":i32[], "svalue":string[]})
      n166 = Unbundle(w241) -> ("lvalue"=w240:i32[], "svalue"=w239:string[])
      "[i32][String] example" <- w243
    }
    frame #2 {
      n167 = local read "Argin (lvalue)"() -> (w248:i32[])
      n168 = local read "Argin (svalue)"() -> (w249:string[])
      n169 = Equal?(x=w247, y=w249) -> (x = y?=w251:bool)
      n170 = Equal?(x=w248, y=w246) -> (x = y?=w250:bool)
      n171 = And(x=w250, y=w251) -> (x .and. y?=→"data":bool)
      "Argout (svalue)" <- w247
      "Argout (lvalue)" <- w246
    }
  }
  n172 = call "RandomArray.vi"("random array size"=16, "factor"=10.0) -> ("random array"=w180:dbl[])
  n173 = for {
    N: 12 -> [_]
    tunnel: [w253] -> w75 mode=indexing
    n174 = call "RandomArray.vi"("random array size"=16, "factor"=10.0) -> ("random array"=w257:dbl[])
    n175 = To Unsigned Byte Integer(number=w257) -> (unsigned 8bit integer=w256:u8[])
    n176 = Byte Array To String(unsigned byte array=w256) -> (string=w253:string)
  }
  "Argin" <- w75
  n177 = To Unsigned Byte Integer(number=w180) -> (unsigned 8bit integer=w94:u8[])
  n178 = Byte Array To String(unsigned byte array=w94) -> (string=w86:string)
  "Argin" <- w86
  n179 = call-poly "_Argin.vi"("argin"=w86) -> ("ArgIO"=w184:cluster{"num data":u8[], "str data":string[]})
  n180 = local read "TangoTest Device Name"() -> (w181:string)
  n181 = call "_TangoExecuteCommand.vi"("argin"=w184, "command name"=w182, "device name"=w181) -> ("error out"=w10:errorcluster, "argout"=w183:cluster{"num data":u8[], "str data":string[]})  [unwired: 1 in]
  n182 = Unbundle By Name(w10) -> ("status"=w11:bool)
  n183 = Not(x=w11) -> (.not. x?=→"cmd":bool)
  n184 = call-poly "_Argout.vi"("ArgIO"=w183) -> ("argout"=w85:string)
  "Argout" <- w85
  n185 = call-poly "_Argin.vi"("argin"=w75) -> ("ArgIO"=w78:cluster{"num data":u8[], "str data":string[]})
  n186 = local read "TangoTest Device Name"() -> (w81:string)
  n187 = call "_TangoExecuteCommand.vi"("argin"=w78, "command name"=w80, "device name"=w81) -> ("error out"=w6:errorcluster, "argout"=w79:cluster{"num data":u8[], "str data":string[]})  [unwired: 1 in]
  n188 = Equal?(x=w85, y=w86) -> (x = y?=→"data":bool)
  n189 = Unbundle By Name(w6) -> ("status"=w8:bool)
  n190 = call-poly "_Argout.vi"("ArgIO"=w79) -> ("argout"=w76:string[])
  "Argout" <- w76
  n191 = Not(x=w8) -> (.not. x?=→"cmd":bool)
  n192 = Equal?(x=w76, y=w75) -> (x = y?=→"data":bool)
  "[I32] example" <- w190
  "String example" <- w182
  "[i16] example" <- w176
  "[u16] example" <- w168
  "[u32] example" <- w157
  "i16 example" <- w152
  "u16 example" <- w144
  "i32 example" <- w133
  "u32 example" <- w127
  "SGL example" <- w116
  "DBL example" <- w113
  "[SGL] example" <- w107
  "[DBL] example" <- w98
  "[u8] example" <- w88
  "[String] example" <- w80
  "TF example" <- w70
  "Void Example" <- w59
